vi "操作日志.vi"(8 "error in (no error)":errorcluster, 11 "日志信息":string) -> (0 "error out":errorcluster)   [LabVIEW 2016, in "斯坦道多参数.lvlib"]
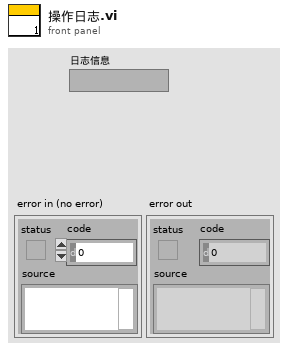
[diagram p1: front panel]
types:
  T1 = typedef "操作日志字段定义.ctl" = cluster{"时间":timestamp, "参数":string, "日志信息":string, "流程参数":string}
  T2 = typedef "数据库类型.ctl" = enum16{"Access", "SQLite"}
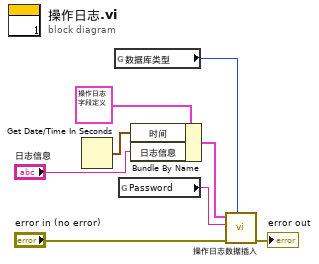
[diagram p0: block diagram]
diagram:
  n1 = Get Date/Time In Seconds() -> (seconds since 1Jan1904=w3:timestamp)
  n2 = global read "断电保存变量.vi" "数据库类型"() -> (w6:T2)
  n3 = global read "断电保存变量.vi" "Password"() -> (w1:string)
  n4 = Bundle By Name(cluster=T1 {"时间"=timestamp(0 s since 1904-01-01), "参数"="多参数", "日志信息"="", "流程参数"=""} ("data"), "时间"=w3, "日志信息"="日志信息") -> (w4:T1)
  n5 = call "操作日志数据插入.vi"("data"=w4, "Password"=w1, "错误输入（无错误）"="error in (no error)", "数据库类型"=w6) -> ("错误输出"=→"error out":errorcluster)  [unwired: 6 in]
